vi "2L08_lit_tableur.vi"(11 "Chemin src*.csv":path caption="chemin src*.csv") -> (1 "dN(t)":dbl[](array[numeric]), 2 "t":dbl[](array[numeric]), 3 "Données":dbl[][](array[numeric]) caption="Données 2D" format="%0.3f")   [LabVIEW 2010, in "lv_02.lvlib"]
doc: "Lire le contenu d'un fichier CSV (données spécifiques FMD) afin de disposer de 2 tableaux 1D contenant le temps t et le nombre de défaillances dN(t)."
uses:
  lv_02.lvlib
  <vilib>/Utility/file.llb/Read From Spreadsheet File (DBL).vi
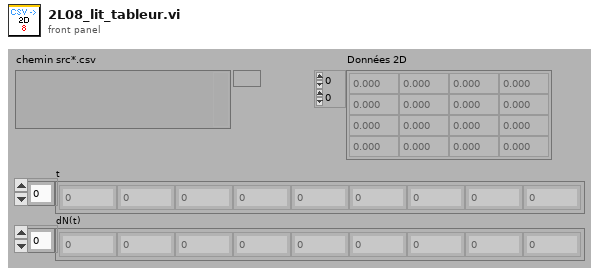
[diagram p1: front panel]
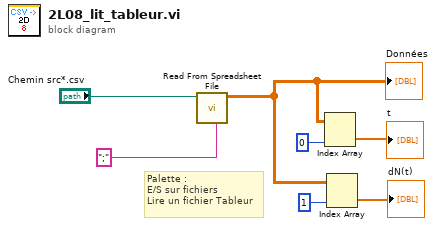
[diagram p0: block diagram]
diagram:
  # "Palette : \nE/S sur fichiers\nLire un fichier Tableur"
  n1 = call-poly <vilib>:"Read From Spreadsheet File.vi"("delimiter (\\t)"=";" ("delimiter (\\t)"), "file path (dialog if empty)"="Chemin src*.csv") -> ("all rows"=w3:dbl[][])  [unwired: 5 in, 4 out]
  "Données" <- w3
  n2 = Index Array(array=w3, index (col)=0 ("indice désactivé (col)")) -> (element=→"t":dbl[])  [unwired: 1 in]
  n3 = Index Array(array=w3, index (col)=1 ("indice désactivé (col)")) -> (element=→"dN(t)":dbl[])  [unwired: 1 in]
